vi "UA_XML Get Server config info.vi"(1 "xml Raw Data":string[](array[string])) -> (0 "Server config info":T1)   [LabVIEW 2013]
uses:
  UA_Server config info.ctl
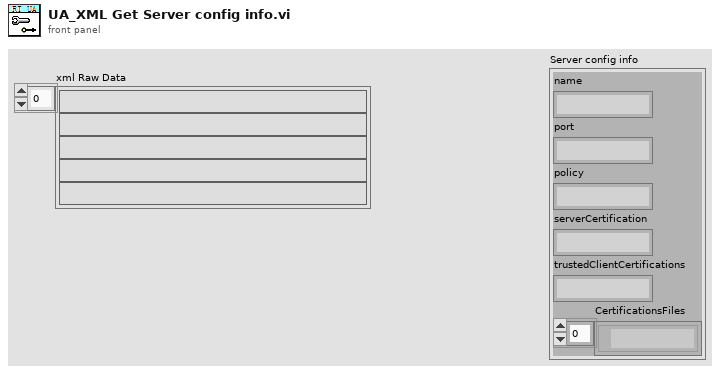
[diagram p1: front panel]
types:
  T1 = typedef "UA_Server config info.ctl" = cluster{"name":string, "port":string, "policy":string, "serverCertification":string, "trustedClientCertifications":string, "CertificationsFiles":path[]}
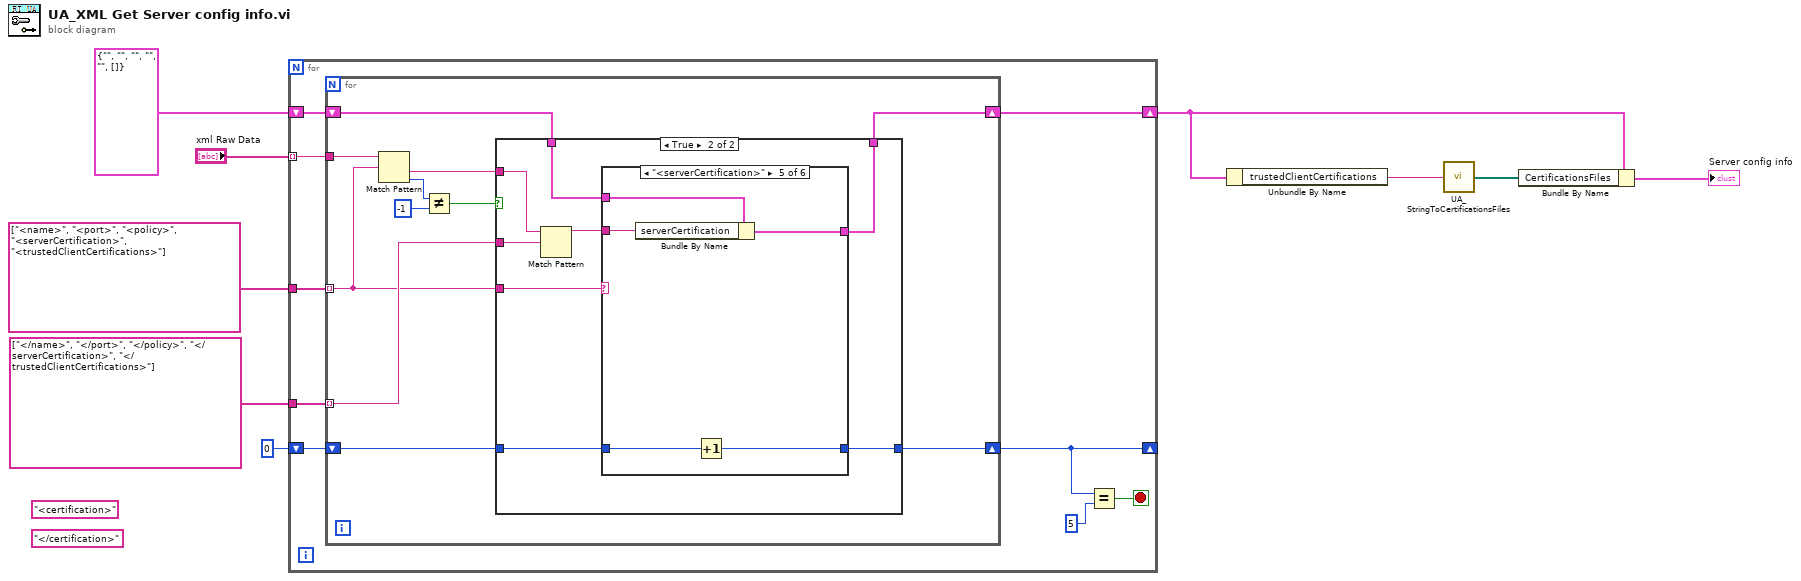
[diagram p0: block diagram]
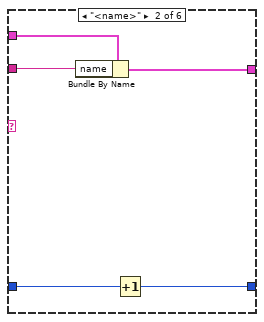
[diagram p4: hidden frame]
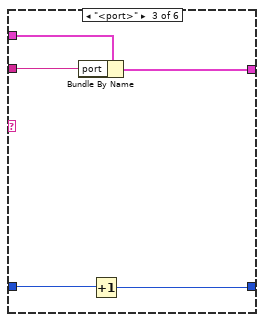
[diagram p5: hidden frame]
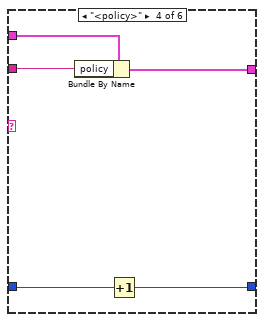
[diagram p6: hidden frame]
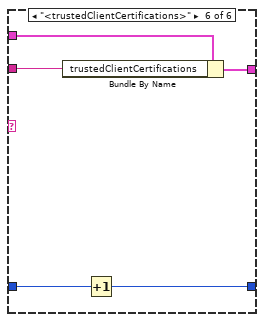
[diagram p7: hidden frame]
diagram:
  (unwired) "<certification>"
  (unwired) "</certification>"
  n1 = for {
    tunnel: "xml Raw Data" -> [w18] mode=indexing
    tunnel: string[] ["<name>", "<port>", "<policy>", "<serverCertification>", "<trustedClientCertifications>"] -> [w17]
    tunnel: string[] ["</name>", "</port>", "</policy>", "</serverCertification>", "</trustedClientCertifications>"] -> [w16]
    shift-right: [w14] -> w4
    shift-left: T1 {"name"="", "port"="", "policy"="", "serverCertification"="", "trustedClientCertifications"="", "CertificationsFiles"=[]} ("Server config info") -> [w15]
    shift-right: [w12] -> _
    shift-left: 0 -> [w13]
    stop <- w10 stop-if-true
    n2 = for {
      tunnel: w18 -> [w29]
      tunnel: w17 -> [w21] mode=indexing
      tunnel: w16 -> [w24] mode=indexing
      shift-right: [w22] -> w14
      shift-left: w15 -> [w23]
      shift-right: [w19] -> w12
      shift-left: w13 -> [w20]
      n3 = Match Pattern(string=w29, regular expression=w21) -> (after substring=w25:string, offset past match=w28:i32)  [unwired: 1 in, 2 out]
      n4 = Not Equal?(x=w28, y=-1) -> (x != y?=w26:bool)
      n5 = case shown="True" w26 {
        tunnel: w25 -> [_ w39]
        tunnel: w24 -> [_ w38]
        tunnel: w23 -> [w31 w37]
        tunnel: [w31 w35] -> w22
        tunnel: w21 -> [_ w34]
        tunnel: w20 -> [w30 w33]
        tunnel: [w30 w32] -> w19
        frame False {
        }
        frame True {
          n6 = Match Pattern(string=w39, regular expression=w38) -> (before substring=w36:string)  [unwired: 1 in, 3 out]
          n7 = case shown="\"<serverCertification>\"" w34 {
            tunnel: w37 -> [w41 w46 w51 w56 w61 w66]
            tunnel: w36 -> [_ w45 w50 w55 w60 w65]
            tunnel: [w41 w44 w49 w54 w59 w64] -> w35
            tunnel: w33 -> [w40 w43 w48 w53 w58 w63]
            tunnel: [w40 w42 w47 w52 w57 w62] -> w32
            frame "假", Default {
            }
            frame "<name>" {
              n8 = Bundle By Name(cluster=w46, "name"=w45) -> (w44:T1)
              n9 = Increment(x=w43) -> (x+1=w42:i32)
            }
            frame "<port>" {
              n10 = Bundle By Name(cluster=w51, "port"=w50) -> (w49:T1)
              n11 = Increment(x=w48) -> (x+1=w47:i32)
            }
            frame "<policy>" {
              n12 = Bundle By Name(cluster=w56, "policy"=w55) -> (w54:T1)
              n13 = Increment(x=w53) -> (x+1=w52:i32)
            }
            frame "<serverCertification>" {
              n14 = Bundle By Name(cluster=w61, "serverCertification"=w60) -> (w59:T1)
              n15 = Increment(x=w58) -> (x+1=w57:i32)
            }
            frame "<trustedClientCertifications>" {
              n16 = Bundle By Name(cluster=w66, "trustedClientCertifications"=w65) -> (w64:T1)
              n17 = Increment(x=w63) -> (x+1=w62:i32)
            }
          }
        }
      }
    }
    n18 = Equal?(x=w12, y=5) -> (x = y?=w10:bool)
  }
  n19 = Unbundle By Name(w4) -> ("trustedClientCertifications"=w1:string)
  n20 = call "UA_StringToCertificationsFiles.vi"("Cerfitications String"=w1) -> ("file"=w2:path[])
  n21 = Bundle By Name(cluster=w4, "CertificationsFiles"=w2) -> (→"Server config info":T1)
